vi "simple fish4.vi"(8 "pointer length":dbl=20.0, 9 "orientation":dbl, 10 "y":dbl, 11 "x":dbl) -> (3 "XY Graph":cluster{dbl[], dbl[]}[](graph))   [LabVIEW 2012]
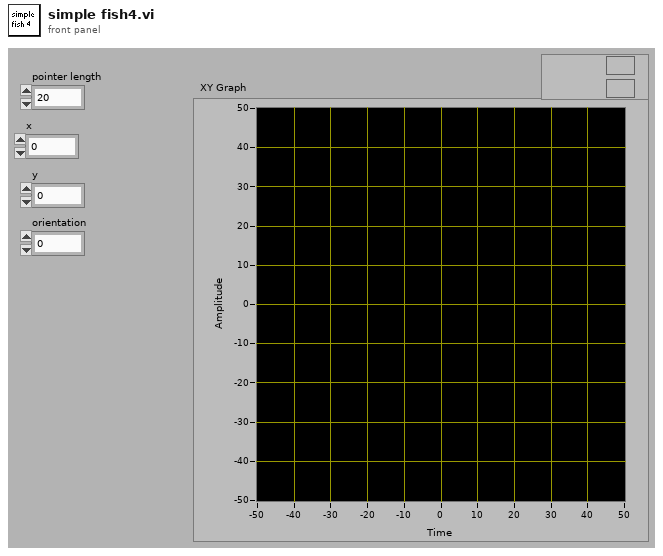
[diagram p1: front panel]
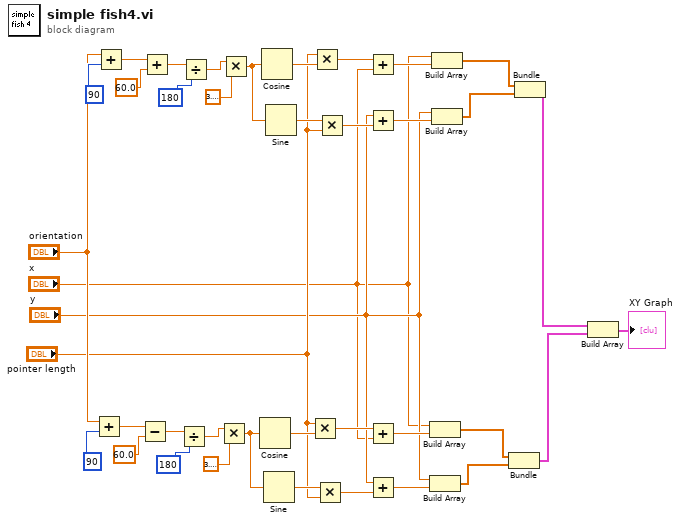
[diagram p0: block diagram]
diagram:
  n1 = Add(x="orientation", y=90) -> (x+y=w17:dbl)
  n2 = Add(x="orientation", y=90) -> (x+y=w26:dbl)
  n3 = Subtract(x=w17, y=60.0) -> (x-y=w19:dbl)
  n4 = Add(x=w26, y=60.0) -> (x+y=w24:dbl)
  n5 = Divide(x=w19, y=180) -> (x/y=w9:dbl)
  n6 = Divide(x=w24, y=180) -> (x/y=w36:dbl)
  n7 = Multiply(x=w9, y=3.141592653589793) -> (x*y=w11:dbl)
  n8 = Multiply(x=w36, y=3.141592653589793) -> (x*y=w32:dbl)
  n9 = Cosine(x=w11) -> (cos(x)=w13:dbl)
  n10 = Cosine(x=w32) -> (cos(x)=w30:dbl)
  n11 = Sine(x=w11) -> (sin(x)=w14:dbl)
  n12 = Sine(x=w32) -> (sin(x)=w29:dbl)
  n13 = Multiply(x="pointer length", y=w13) -> (x*y=w12:dbl)
  n14 = Multiply(x="pointer length", y=w30) -> (x*y=w31:dbl)
  n15 = Multiply(x=w14, y="pointer length") -> (x*y=w16:dbl)
  n16 = Multiply(x=w29, y="pointer length") -> (x*y=w27:dbl)
  n17 = Add(x=w31, y="x") -> (x+y=w23:dbl)
  n18 = Add(x="y", y=w27) -> (x+y=w22:dbl)
  n19 = Add(x=w12, y="x") -> (x+y=w20:dbl)
  n20 = Add(x="y", y=w16) -> (x+y=w21:dbl)
  n21 = Build Array("x", w20) -> (w4:dbl[])
  n22 = Build Array("y", w21) -> (w5:dbl[])
  n23 = Build Array("x", w23) -> (w33:dbl[])
  n24 = Build Array("y", w22) -> (w34:dbl[])
  n25 = Bundle(w4, w5) -> (w1:cluster{dbl[], dbl[]})  [unwired: 1 in]
  n26 = Bundle(w33, w34) -> (w39:cluster{dbl[], dbl[]})  [unwired: 1 in]
  n27 = Build Array(w39, w1) -> (→"XY Graph":cluster{dbl[], dbl[]}[])
